vi "Get EUI Events.vi"(8 "error in (no error)":errorcluster, 11 "EUI Events in":refnum<class "EUI Events.lvclass">) -> (0 "error out":errorcluster, 2 "EUI Events":T1, 3 "EUI Events out":refnum<class "EUI Events.lvclass">)   [LabVIEW 2016, in "EUI Events.lvclass"]
uses:
  EUI Events.lvclass
  Typedefs/EUI Events.ctl
  Typedefs/MessageContainer.ctl
  EUI Events.lvclass/EUI Events.ctl
  Typedefs/M1M3SupportEUI_TypeDefs.lvlib
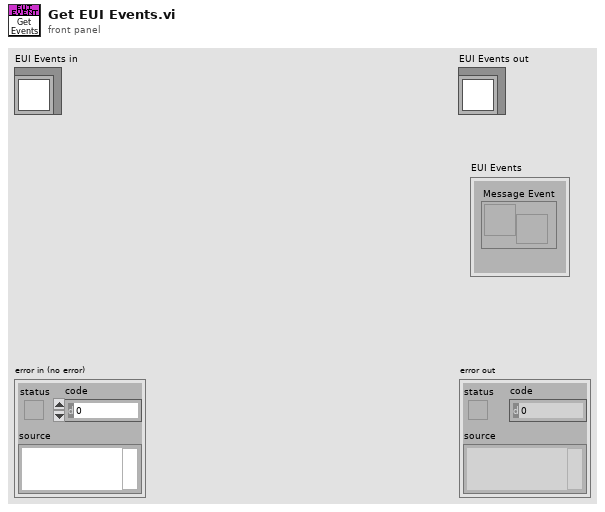
[diagram p1: front panel]
types:
  T1 = typedef "M1M3SupportEUI_TypeDefs.lvlib/EUI Events.ctl" = cluster{"Message Event":refnum<user-event>}
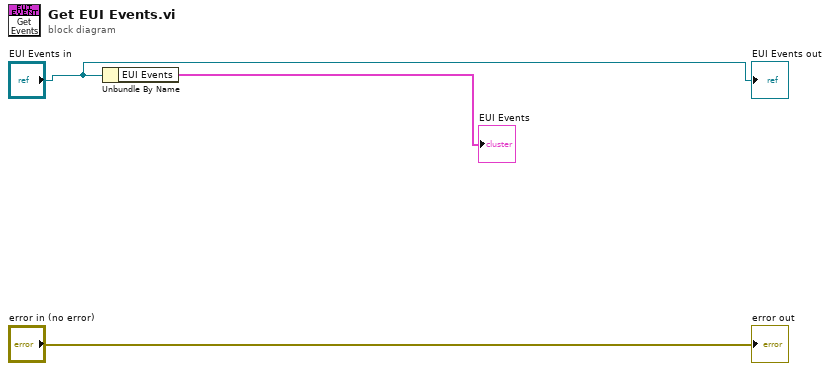
[diagram p0: block diagram]
diagram:
  n1 = Unbundle By Name("EUI Events in") -> ("EUI Events"=→"EUI Events":T1)
  "error out" <- "error in (no error)"
  "EUI Events out" <- "EUI Events in"
